vi "makeDecisions.vi"(8 "error in (no error)":errorcluster, 10 "model":refnum<class "Model.lvclass">, 11 "PausingState in":refnum<class "PausingState.lvclass">) -> (0 "error out":errorcluster, 2 "model 2":refnum<class "Model.lvclass">, 3 "PausingState out":refnum<class "PausingState.lvclass">)   [LabVIEW 2013, in "PausingState.lvclass"]
uses:
  PausingState.lvclass
  Model/Model/Model.lvclass
  ExecutingCycleState/ExecutingCycleState.lvclass
  Typedefs/StateSelector.ctl
  Typedefs/FAMTTypedefs.lvlib
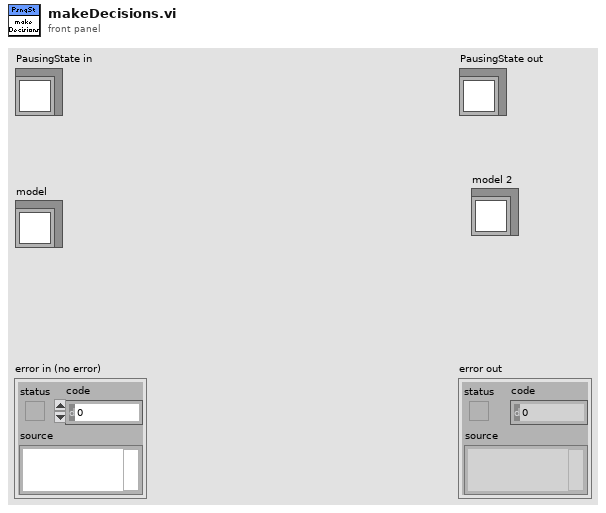
[diagram p1: front panel]
types:
  T1 = typedef "FAMTTypedefs.lvlib/StateSelector.ctl" = enum16{"EndingCycleState", "FaultState", "InteractiveMotionState", "MovingToNewForceState", "OffState", "PausingState", "StandbyState", "StoppedState"}
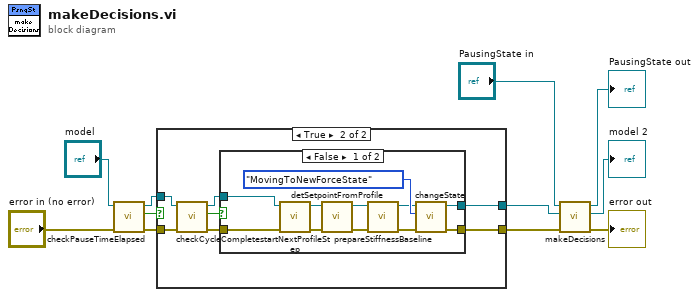
[diagram p0: block diagram]
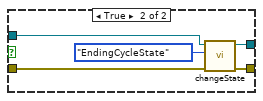
[diagram p3: hidden frame]
diagram:
  n1 = call "checkPauseTimeElapsed.vi"("error in (no error)"="error in (no error)", "Model in"="model") -> ("error out"=w2:errorcluster, "pauseTimeHasElapsedIsTrue"=w7:bool, "Model out"=w5:refnum<class "Model.lvclass">)  [unwired: 7 in]
  n2 = case shown="True" w7 {
    tunnel: w5 -> [w13 w20]
    tunnel: [w13 w18] -> w4
    tunnel: w2 -> [w12 w17]
    tunnel: [w12 w14] -> w1
    frame False {
    }
    frame True {
      n3 = call "checkCycleComplete.vi"("error in (no error)"=w17, "Model in"=w20) -> ("error out"=w16:errorcluster, "cycleCompleteIsTrue"=w15:bool, "Model out"=w19:refnum<class "Model.lvclass">)  [unwired: 7 in]
      n4 = case shown="False" w15 {
        tunnel: w19 -> [w30 w35]
        tunnel: [w29 w34] -> w18
        tunnel: w16 -> [w28 w33]
        tunnel: [w27 w32] -> w14
        frame False {
          n5 = call "startNextProfileStep.vi"("error in (no error)"=w28, "Model in"=w30) -> ("error out"=w25:errorcluster, "Model out"=w26:refnum<class "Model.lvclass">)  [unwired: 8 in]
          n6 = call "detSetpointFromProfile.vi"("error in (no error)"=w25, "Model in"=w26) -> ("error out"=w21:errorcluster, "Model out"=w24:refnum<class "Model.lvclass">)  [unwired: 8 in]
          n7 = call "prepareStiffnessBaseline.vi"("error in (no error)"=w21, "Model in"=w24) -> ("error out"=w22:errorcluster, "Model out"=w23:refnum<class "Model.lvclass">)  [unwired: 8 in]
          n8 = call "changeState.vi"("error in (no error)"=w22, "State:"=StateSelector."MovingToNewForceState", "Model in"=w23) -> ("error out"=w27:errorcluster, "Model out"=w29:refnum<class "Model.lvclass">)  [unwired: 7 in]
        }
        frame True {
          n9 = call "changeState.vi"("error in (no error)"=w33, "State:"=StateSelector."EndingCycleState", "Model in"=w35) -> ("error out"=w32:errorcluster, "Model out"=w34:refnum<class "Model.lvclass">)  [unwired: 7 in]
        }
      }
    }
  }
  n10 = call-parent "makeDecisions.vi"("error in (no error)"=w1, "model"=w4, "EnabledState in"="PausingState in") -> ("error out"=→"error out":errorcluster, "model 2"=→"model 2":refnum<class "Model.lvclass">, "EnabledState out"=→"PausingState out":refnum<class "PausingState.lvclass">)  [unwired: 6 in]
